vi "Open FlexLogger Project.vi"(6 "Timeout(ms)":i32=-1, 8 "error in (no error)":errorcluster, 10 "FlexLoggerProjPath in":path, 11 "FlexLogger_gRPCAPI in":refnum<class "FlexLogger_gRPC.lvclass">) -> (0 "error out":errorcluster, 2 "Timedout?":bool, 3 "FlexLogger_gRPCAPI out":refnum<class "FlexLogger_gRPC.lvclass">)   [LabVIEW 2020, in "FlexLogger_gRPC.lvlib" / "FlexLogger_gRPC.lvclass"]
uses:
  FlexLogger_gRPC.lvclass
  FlexLogger_client/RPC Messages/flexlogger_OpenProjectRequest.ctl
  FlexLogger_gRPC.lvclass/FlexLogger_gRPC.ctl
  FlexLogger_client/FlexLogger_client.lvlib
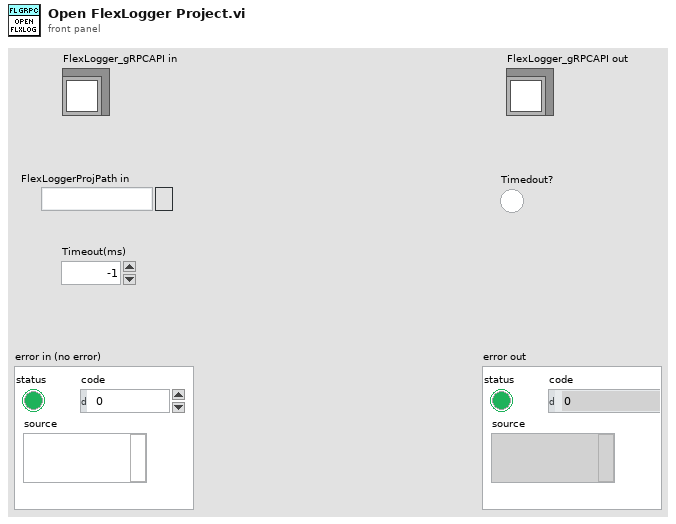
[diagram p1: front panel]
types:
  T1 = typedef "FlexLogger_client.lvlib/flexlogger_OpenProjectRequest.ctl" = cluster{"project_path":string}
  T2 = typedef "grpc-lvsupport-release.lvlib/grpcId.ctl" = u64
  T3 = typedef "FlexLogger_client.lvlib/flexlogger_OpenProjectResponse.ctl" = cluster{"project":T4}
  T4 = typedef "FlexLogger_client.lvlib/flexlogger_ProjectIdentifier.ctl" = cluster{"project_id":string}
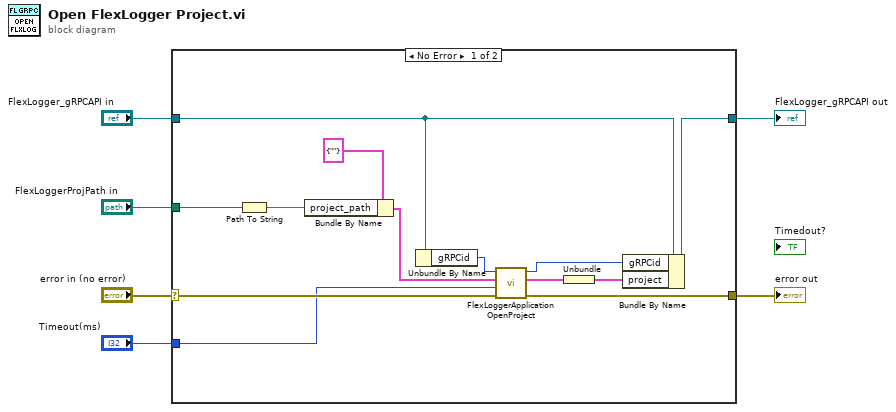
[diagram p0: block diagram]
diagram:
  n1 = case shown="No Error" "error in (no error)" {
    selector: "error in (no error)" -> [w19 w20]
    tunnel: [w18 w20] -> w5
    tunnel: "Timeout(ms)" -> [w17 _]
    tunnel: "FlexLoggerProjPath in" -> [w15 _]
    tunnel: "FlexLogger_gRPCAPI in" -> [w10 w21]
    tunnel: [w9 w21] -> w1
    frame No Error {
      n2 = Path To String(path=w15) -> (string=w14:string)
      n3 = Bundle By Name(cluster=T1 {"project_path"=""} ("Request Data"), "project_path"=w14) -> (w13:T1)
      n4 = Unbundle By Name(w10) -> ("gRPCid"=w12:T2)
      n5 = call "FlexLoggerApplication OpenProject.vi"("error in"=w19, "timeout (ms)"=w17, "Request Data"=w13, "gRPC ID"=w12) -> ("error out"=w18:errorcluster, "Response Data"=w8:T3, "gRPC ID out"=w11:T2)  [unwired: 5 in]
      n6 = Unbundle(w8) -> ("project"=w7:T4)
      n7 = Bundle By Name(cluster=w10, "gRPCid"=w11, "project"=w7) -> (w9:refnum<class "FlexLogger_gRPC.lvclass">)
    }
    frame Error {
    }
  }
  "error out" <- w5
  "FlexLogger_gRPCAPI out" <- w1
